vi "Expert Mode.vi"() -> ()   [LabVIEW 2019]
uses:
  <vilib>/Instr/_visa.llb/VISA Configure Serial Port (Instr).vi
  <vilib>/regexp/Match Regular Expression.xnode
panel:
  in  "Write to File":bool
  in  "Pump Pressure":dbl
  in  "sMDT Code":string
  out "Status":string
  out "Test Passed":bool
  in  "Start":bool
  out "Leak":string
  out "Pressure (mTorr)":dbl
  out "System Information":string
  in  "VISA resource name":refnum<visa-resource-name>="COM1"
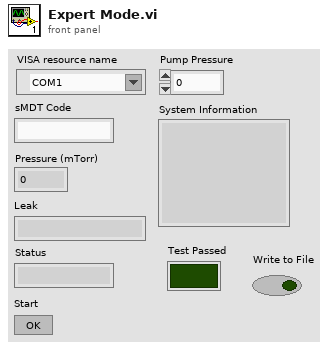
[diagram p1: front panel]
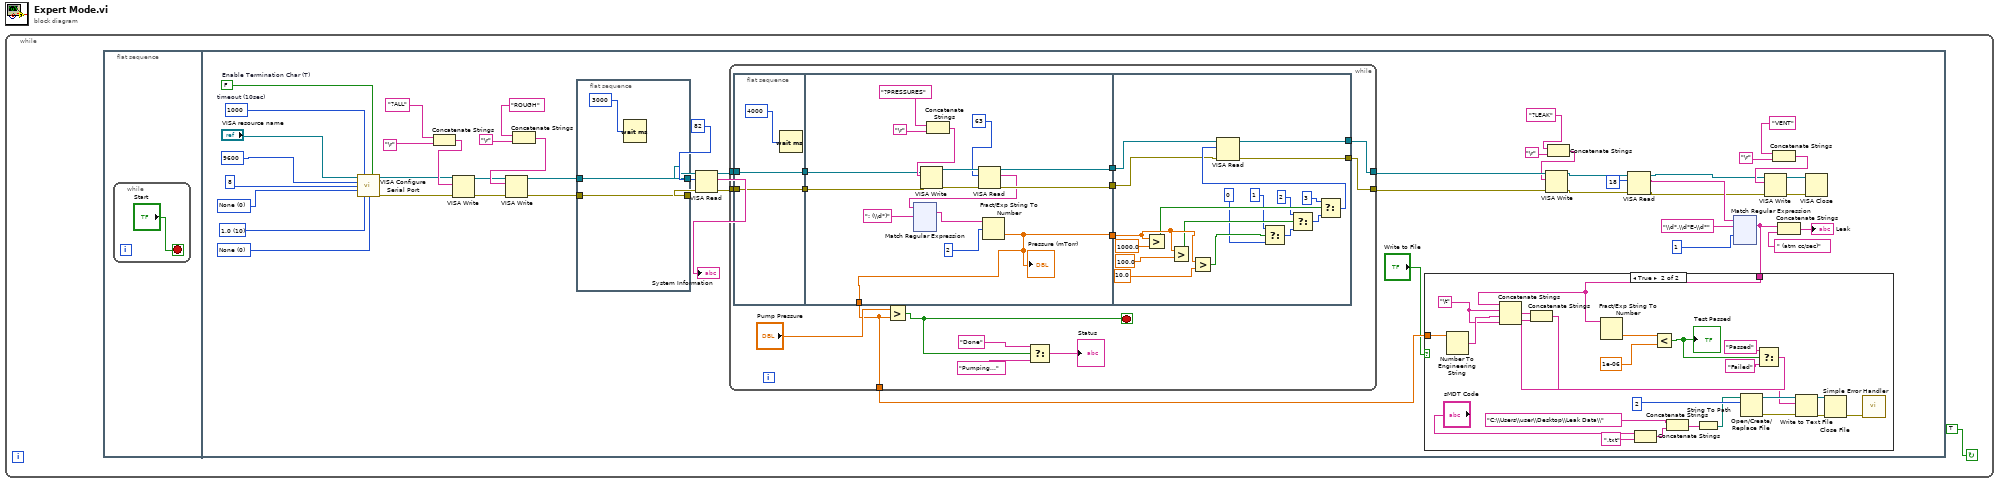
[diagram p0: block diagram]
diagram:
  n1 = while {
    stop <- TRUE continue-if-true
    n2 = flat-sequence {
      frame #0 {
        n3 = while {
          stop <- "Start" stop-if-true
        }
      }
      frame #1 {
        w39 = u16 0 items=["None"=0, "XON/XOFF"=1, "RTS/CTS"=2, "DTR/DSR"=4] ("flow control")
        w40 = u16 10 items=["1.0"=10, "1.5"=15, "2.0"=20] ("stop bits")
        w41 = u16 0 items=["None", "Odd", "Even", "Mark", "Space"] ("parity")
        w49 = FALSE  # Enable Termination Char (T)
        w50 = u32 1000  # timeout (10sec)
        n4 = call-poly "VISA Configure Serial Port"("VISA resource name"="VISA resource name", "timeout (10sec)"=w50, "Enable Termination\nChar (T)"=w49, "baud rate (9600)"=u32 9600 ("baud rate"), "data bits (8)"=u16 8 ("data bits"), "parity (0:none)"=w41, "stop bits (10: 1 bit)"=w40, "flow control (0:none)"=w39) -> ("VISA resource name out"=w45:refnum<visa-resource-name>, "error out"=w44:errorcluster)  [unwired: 6 in]
        n5 = Concatenate Strings("?ALL", "\r") -> (w47:string)
        n6 = VISA Write(VISA resource name=w45, write buffer=w47, error in (no error)=w44) -> (VISA resource name out=w19:refnum<visa-resource-name>, error out=w18:errorcluster)  [unwired: 1 out]
        n7 = Concatenate Strings("ROUGH", "\r") -> (w36:string)
        n8 = VISA Write(VISA resource name=w19, write buffer=w36, error in (no error)=w18) -> (VISA resource name out=w30:refnum<visa-resource-name>, error out=w29:errorcluster)  [unwired: 1 out]
        n9 = flat-sequence {
          tunnel: w30 -> [w355]
          tunnel: w29 -> [w356]
          tunnel: [w356] -> w26
          tunnel: [w355] -> w27
          frame #0 {
            n10 = Wait (ms)(milliseconds to wait=3000) -> ()  [unwired: 1 out]
          }
        }
        n11 = VISA Read(VISA resource name=w27, byte count=82, error in (no error)=w26) -> (VISA resource name out=w24:refnum<visa-resource-name>, read buffer=→"System Information":string, error out=w25:errorcluster)  [unwired: 1 out]
        n12 = while {
          tunnel: w24 -> [w90]
          tunnel: w25 -> [w89]
          tunnel: [w77] -> w12
          tunnel: [w76] -> w11
          tunnel: [w81] -> w10
          stop <- w83 stop-if-true
          n13 = flat-sequence {
            tunnel: w90 -> [w93]
            tunnel: w89 -> [w92]
            tunnel: [w93] -> w88
            tunnel: [w92] -> w87
            tunnel: w88 -> [w102]
            tunnel: w87 -> [w101]
            tunnel: [w94] -> w81
            tunnel: [w99] -> w80
            tunnel: [w100] -> w79
            tunnel: [w94] -> w78
            tunnel: w80 -> [w226]
            tunnel: w79 -> [w227]
            tunnel: w78 -> [w238]
            tunnel: [w225] -> w77
            tunnel: [w224] -> w76
            frame #0 {
              n14 = Wait (ms)(milliseconds to wait=4000) -> ()  [unwired: 1 out]
            }
            frame #1 {
              n15 = Concatenate Strings("?PRESSURES", "\r") -> (w103:string)
              n16 = VISA Write(VISA resource name=w102, write buffer=w103, error in (no error)=w101) -> (VISA resource name out=w108:refnum<visa-resource-name>, error out=w107:errorcluster)  [unwired: 1 out]
              n17 = VISA Read(VISA resource name=w108, byte count=63, error in (no error)=w107) -> (VISA resource name out=w100:refnum<visa-resource-name>, read buffer=w96:string, error out=w99:errorcluster)  [unwired: 1 out]
              n18 = xnode "Match Regular Expression"("input string"=w96, "regular expression"=": (\\d*)") -> ("whole match"=w98:string)  [unwired: 4 in, 4 out]
              n19 = Fract/Exp String To Number(string=w98, offset=2) -> (number=w94:dbl)  [unwired: 2 in, 1 out]
              "Pressure (mTorr)" <- w94
            }
            frame #2 {
              n20 = Greater?(x=w238, y=1000.0) -> (0:w234:bool)
              n21 = Greater?(x=w238, y=100.0) -> (0:w233:bool)
              n22 = Greater?(x=w238, y=10.0) -> (0:w232:bool)
              n23 = Select(t=1, s=w232, f=0) -> (s? t:f=w240:i32)
              n24 = Select(t=2, s=w233, f=w240) -> (s? t:f=w239:i32)
              n25 = Select(t=3, s=w234, f=w239) -> (s? t:f=w228:i32)
              n26 = VISA Read(VISA resource name=w227, byte count=w228, error in (no error)=w226) -> (VISA resource name out=w225:refnum<visa-resource-name>, error out=w224:errorcluster)  [unwired: 2 out]
            }
          }
          n27 = Greater?(x="Pump Pressure", y=w81) -> (0:w83:bool)
          n28 = Select(t="Done", s=w83, f="Pumping...") -> (s? t:f=→"Status":string)
        }
        n29 = Concatenate Strings("?LEAK", "\r") -> (w7:string)
        n30 = VISA Write(VISA resource name=w12, write buffer=w7, error in (no error)=w11) -> (VISA resource name out=w6:refnum<visa-resource-name>, error out=w5:errorcluster)  [unwired: 1 out]
        n31 = VISA Read(VISA resource name=w6, byte count=18, error in (no error)=w5) -> (VISA resource name out=w14:refnum<visa-resource-name>, read buffer=w15:string, error out=w13:errorcluster)  [unwired: 1 out]
        n32 = xnode "Match Regular Expression"("input string"=w15, "regular expression"="\\d*.\\d*E-\\d*", "offset (0)"=1) -> ("whole match"=w4:string)  [unwired: 3 in, 4 out]
        n33 = case shown="True" "Write to File" {
          tunnel: w10 -> [_ w61]
          tunnel: w4 -> [_ w52]
          frame False {
          }
          frame True {
            w56 = "\t"
            n34 = Number To Engineering String(4:w61) -> (0:w57:string)  [unwired: 3 in]
            n35 = Concatenate Strings(w52, w56, w57, w56) -> (w55:string)
            n36 = Fract/Exp String To Number(string=w52) -> (number=w74:dbl)  [unwired: 3 in, 1 out]
            n37 = Concatenate Strings("sMDT Code", ".txt") -> (w62:string)
            n38 = Less?(x=w74, y=1e-06) -> (x < y?=w60:bool)
            "Test Passed" <- w60
            n39 = Concatenate Strings("C:\\Users\\user\\Desktop\\Leak Data\\", w62) -> (w67:string)
            n40 = String To Path(string=w67) -> (path=w66:path)
            n41 = Open/Create/Replace File(file path (use dialog)=w66, operation (0:open)=2) -> (refnum out=w72:refnum<file>, error out=w70:errorcluster)  [unwired: 4 in, 1 out]
            n42 = Select(t="Passed", s=w60, f="Failed") -> (s? t:f=w54:string)
            n43 = Concatenate Strings(w55, w54) -> (w53:string)
            n44 = Write to Text File(file (use dialog)=w72, text=w53, error in=w70) -> (refnum out=w71:refnum<file>, error out=w69:errorcluster)  [unwired: 1 in, 1 out]
            n45 = Close File(refnum=w71, error in=w69) -> (error out=w68:errorcluster)  [unwired: 1 out]
            n46 = call <vilib>:"Simple Error Handler.vi"("error in (no error)"=w68) -> ()  [unwired: 4 in, 5 out]
          }
        }
        n47 = Concatenate Strings("VENT", "\r") -> (w33:string)
        n48 = VISA Write(VISA resource name=w14, write buffer=w33, error in (no error)=w13) -> (VISA resource name out=w32:refnum<visa-resource-name>, error out=w31:errorcluster)  [unwired: 1 out]
        n49 = Concatenate Strings(w4, " (atm cc/sec)") -> (→"Leak":string)
        n50 = VISA Close(VISA resource name=w32, error in (no error)=w31) -> ()  [unwired: 1 out]
      }
    }
  }
